vi "Write Services.vi"(8 "error in (no error)":errorcluster, 10 "Services":string[](array[string]), 11 "CS++DIMMonitor in":refnum<class "CS++DIMMonitor.lvclass">) -> (0 "error out":errorcluster, 3 "CS++DIMMonitor out":refnum<class "CS++DIMMonitor.lvclass">)   [LabVIEW 2016, in "CS++DIMMonitor.lvlib" / "CS++DIMMonitor.lvclass"]
doc: "Write Services to attribute."
uses:
  CS++DIMMonitor.lvclass
  CS++DIMMonitor.lvclass/CS++DIMMonitor.ctl
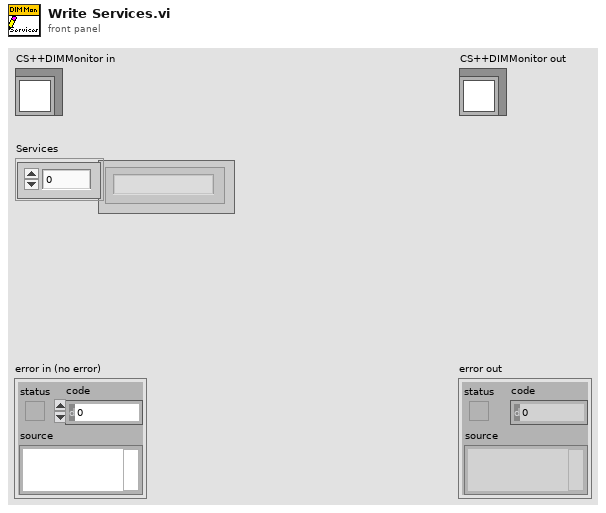
[diagram p1: front panel]
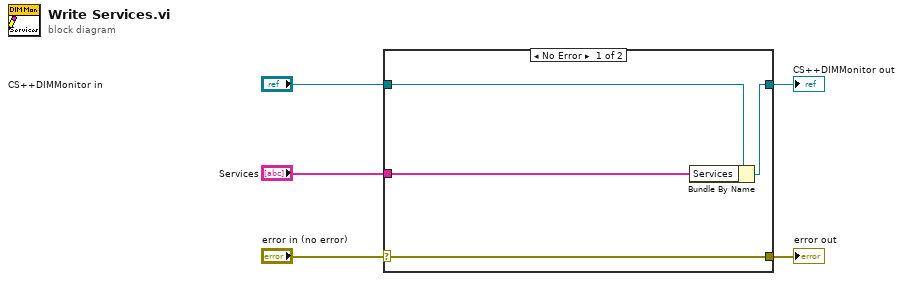
[diagram p0: block diagram]
diagram:
  n1 = case shown="No Error" "error in (no error)" {
    selector: "error in (no error)" -> [w9 w10]
    tunnel: [w9 w10] -> w4
    tunnel: [w7 w11] -> w2
    tunnel: "CS++DIMMonitor in" -> [w8 w11]
    tunnel: "Services" -> [w6 _]
    frame No Error {
      n2 = Bundle By Name(cluster=w8, "Services"=w6) -> (w7:refnum<class "CS++DIMMonitor.lvclass">)
    }
    frame Error {
    }
  }
  "error out" <- w4
  "CS++DIMMonitor out" <- w2
